vi "氨氮通讯.vi"() -> ()   [LabVIEW 2016, in "斯坦道氨氮.lvlib"]
uses:
  <vilib>/NI/Modbus Library/API/Wrapper/Create TCP Slave.vi
  <vilib>/Utility/config.llb/Write Key (String).vi
  <vilib>/Plasmionique/MB Master/MB_Master/MB_Master.lvclass
  <vilib>/NI/Modbus Library/API/slave/Modbus Slave.lvclass
  <vilib>/Utility/config.llb/NI_LVConfig.lvlib
  <vilib>/Plasmionique/MB Master/MB Master.lvlib
  <vilib>/NI/Modbus Library/API/Wrapper/API Main.lvlib
panel:
  out "测量数据区":T1 {"单位" items=["ug/L", "mg/L", "ppm", "mg/m3", "cm", "ppb", "ug/m3", "%", "nmol/mol", "umol/mol", "MPN/L", "MPN/100ml", "ng/m3", "NTU", "无量纲", "ms/cm", "us/cm", "℃", "mV", "万个/L"]}
  out "状态告警区":u16[](array[numeric])
  out "测量数据区":u16[](array[numeric])
  out "序列号":string
  out "状态告警区":T2 {"告警代码" items=["无告警", "缺试剂告警", "缺水样告警", "缺蒸馏水告警", "缺标液告警", "仪表漏液告警", "标定异常告警", "超量程告警", "加热异常", "低试剂预警", "超上限告警", "超下限告警", "仪表内部其他异常", "滴定异常告警", "电极异常告警", "量程切换告警", "参数设置告警", "PH电极电位异常", "电导率电极异常", "浊度光度异常", "溶解氧电极异常", "溶解氧光强异常", "温度异常告警", "PH异常告警", "溶解氧异常告警", "电导率异常告警", "浊度异常告警", "叶绿素异常告警", "藻密度异常告警", "蓝绿藻异常告警", "ORP异常告警", "氨氮异常告警", "清洁刷异常告警", "SD卡异常告警", "蓝牙异常告警", "Wifi异常告警", "流程异常告警"]; "故障代码" items=["无故障", "电机故障", "温度故障", "通讯故障", "滴定故障"]}
  out "status":bool
  out "关键参数区":T3
  in  "读关键参数区":bool
  in  "读状态告警区":bool
  in  "读测量数据区":bool
  in  "站号":u16(ring) items=["总磷"=1, "氨氮"=3]
  in  "停止":bool
  in  "启动":bool
  in  "控制命令":u16(ring) items=["启动测量"=1, "标样核查"=2, "零点核查"=3, "跨度核查"=4, "空白测试"=5, "平行样测试"=6, "加标回收"=7, "空白校准"=8, "标样校准"=9, "初始化（清洗）"=10, "停止测试"=11, "仪器重启"=12, "校时"=13, "模式设置"=14, "测量间隔设置"=15]
  in  "控制命令参数":u16[](array[numeric]) format="%04xH"
  in  "VISA Resource":refnum<visa-resource-name>
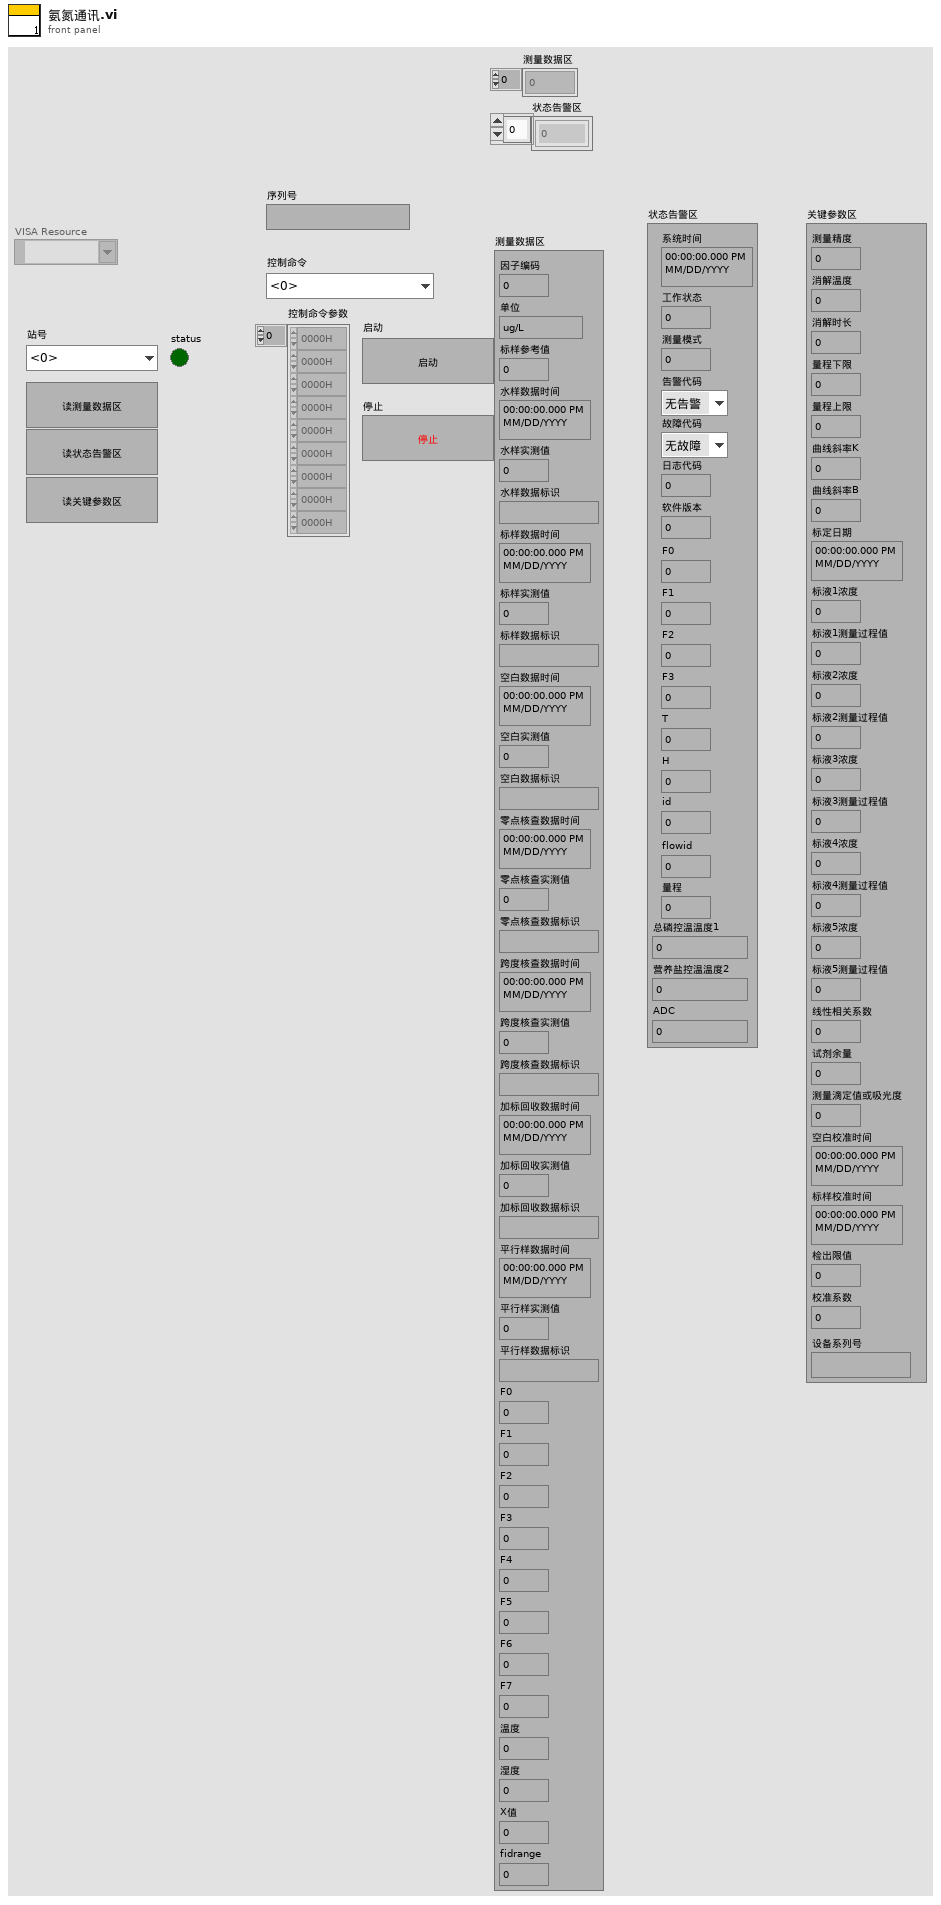
[diagram p1: front panel]
types:
  T1 = cluster{"因子编码":u32, "单位":u16, "标样参考值":sgl, "水样数据时间":timestamp, "水样实测值":sgl, "水样数据标识":string, "标样数据时间":timestamp, "标样实测值":sgl, "标样数据标识":string, "空白数据时间":timestamp, "空白实测值":sgl, "空白数据标识":string, "零点核查数据时间":timestamp, "零点核查实测值":sgl, "零点核查数据标识":string, "跨度核查数据时间":timestamp, "跨度核查实测值":sgl, "跨度核查数据标识":string, "加标回收数据时间":timestamp, "加标回收实测值":sgl, "加标回收数据标识":string, "平行样数据时间":timestamp, "平行样实测值":sgl, "平行样数据标识":string, "F0":sgl, "F1":sgl, "F2":sgl, "F3":sgl, "F4":sgl, "F5":sgl, "F6":sgl, "F7":sgl, "温度":sgl, "湿度":sgl, "X值":sgl, "fidrange":sgl}
  T2 = cluster{"系统时间":timestamp, "工作状态":u16, "测量模式":u16, "告警代码":u16, "故障代码":u16, "日志代码":u16, "软件版本":u16, "F0":sgl, "F1":sgl, "F2":sgl, "F3":sgl, "T":sgl, "H":sgl, "id":u16, "flowid":u16, "量程":u16, "ADC":sgl, "营养盐控温温度2":sgl, "总磷控温温度1":sgl}
  T3 = cluster{"测量精度":u16, "消解温度":u16, "消解时长":u16, "量程下限":sgl, "量程上限":sgl, "曲线斜率K":sgl, "曲线斜率B":sgl, "标定日期":timestamp, "标液1浓度":sgl, "标液1测量过程值":sgl, "标液2浓度":sgl, "标液2测量过程值":sgl, "标液3浓度":sgl, "标液3测量过程值":sgl, "标液4浓度":sgl, "标液4测量过程值":sgl, "标液5浓度":sgl, "标液5测量过程值":sgl, "线性相关系数":sgl, "试剂余量":u32, "测量滴定值或吸光度":sgl, "空白校准时间":timestamp, "标样校准时间":timestamp, "检出限值":sgl, "校准系数":sgl, "设备系列号":string}
  T4 = typedef "NI_LVConfig.lvlib/Config Data RefNum.ctl" = refnum<k1>
  T5 = enum8{"Enabled", "Disabled", "Disabled and Grayed Out"}
  T6 = cluster{"系统时间":timestamp, "工作状态":enum16{"空闲", "水样测试", "标样核查", "零点核查", "跨度核查", "空白测试", "平行样测试", "加标回收", "空白校准", "标样校准", "初始化（清洗）"}, "测量模式":enum16{"待机", "连续模式", "周期模式", "定点模式", "受控模式", "手动模式"}, "告警代码":u16, "故障代码":u16, "日志代码":u16, "软件版本":u16, "F0":sgl, "F1":sgl, "F2":sgl, "F3":sgl, "T":sgl, "H":sgl, "id":u16, "flowid":u16, "量程":u16, "总磷控温温度1":sgl, "营养盐控温温度2":sgl, "ADC":sgl}
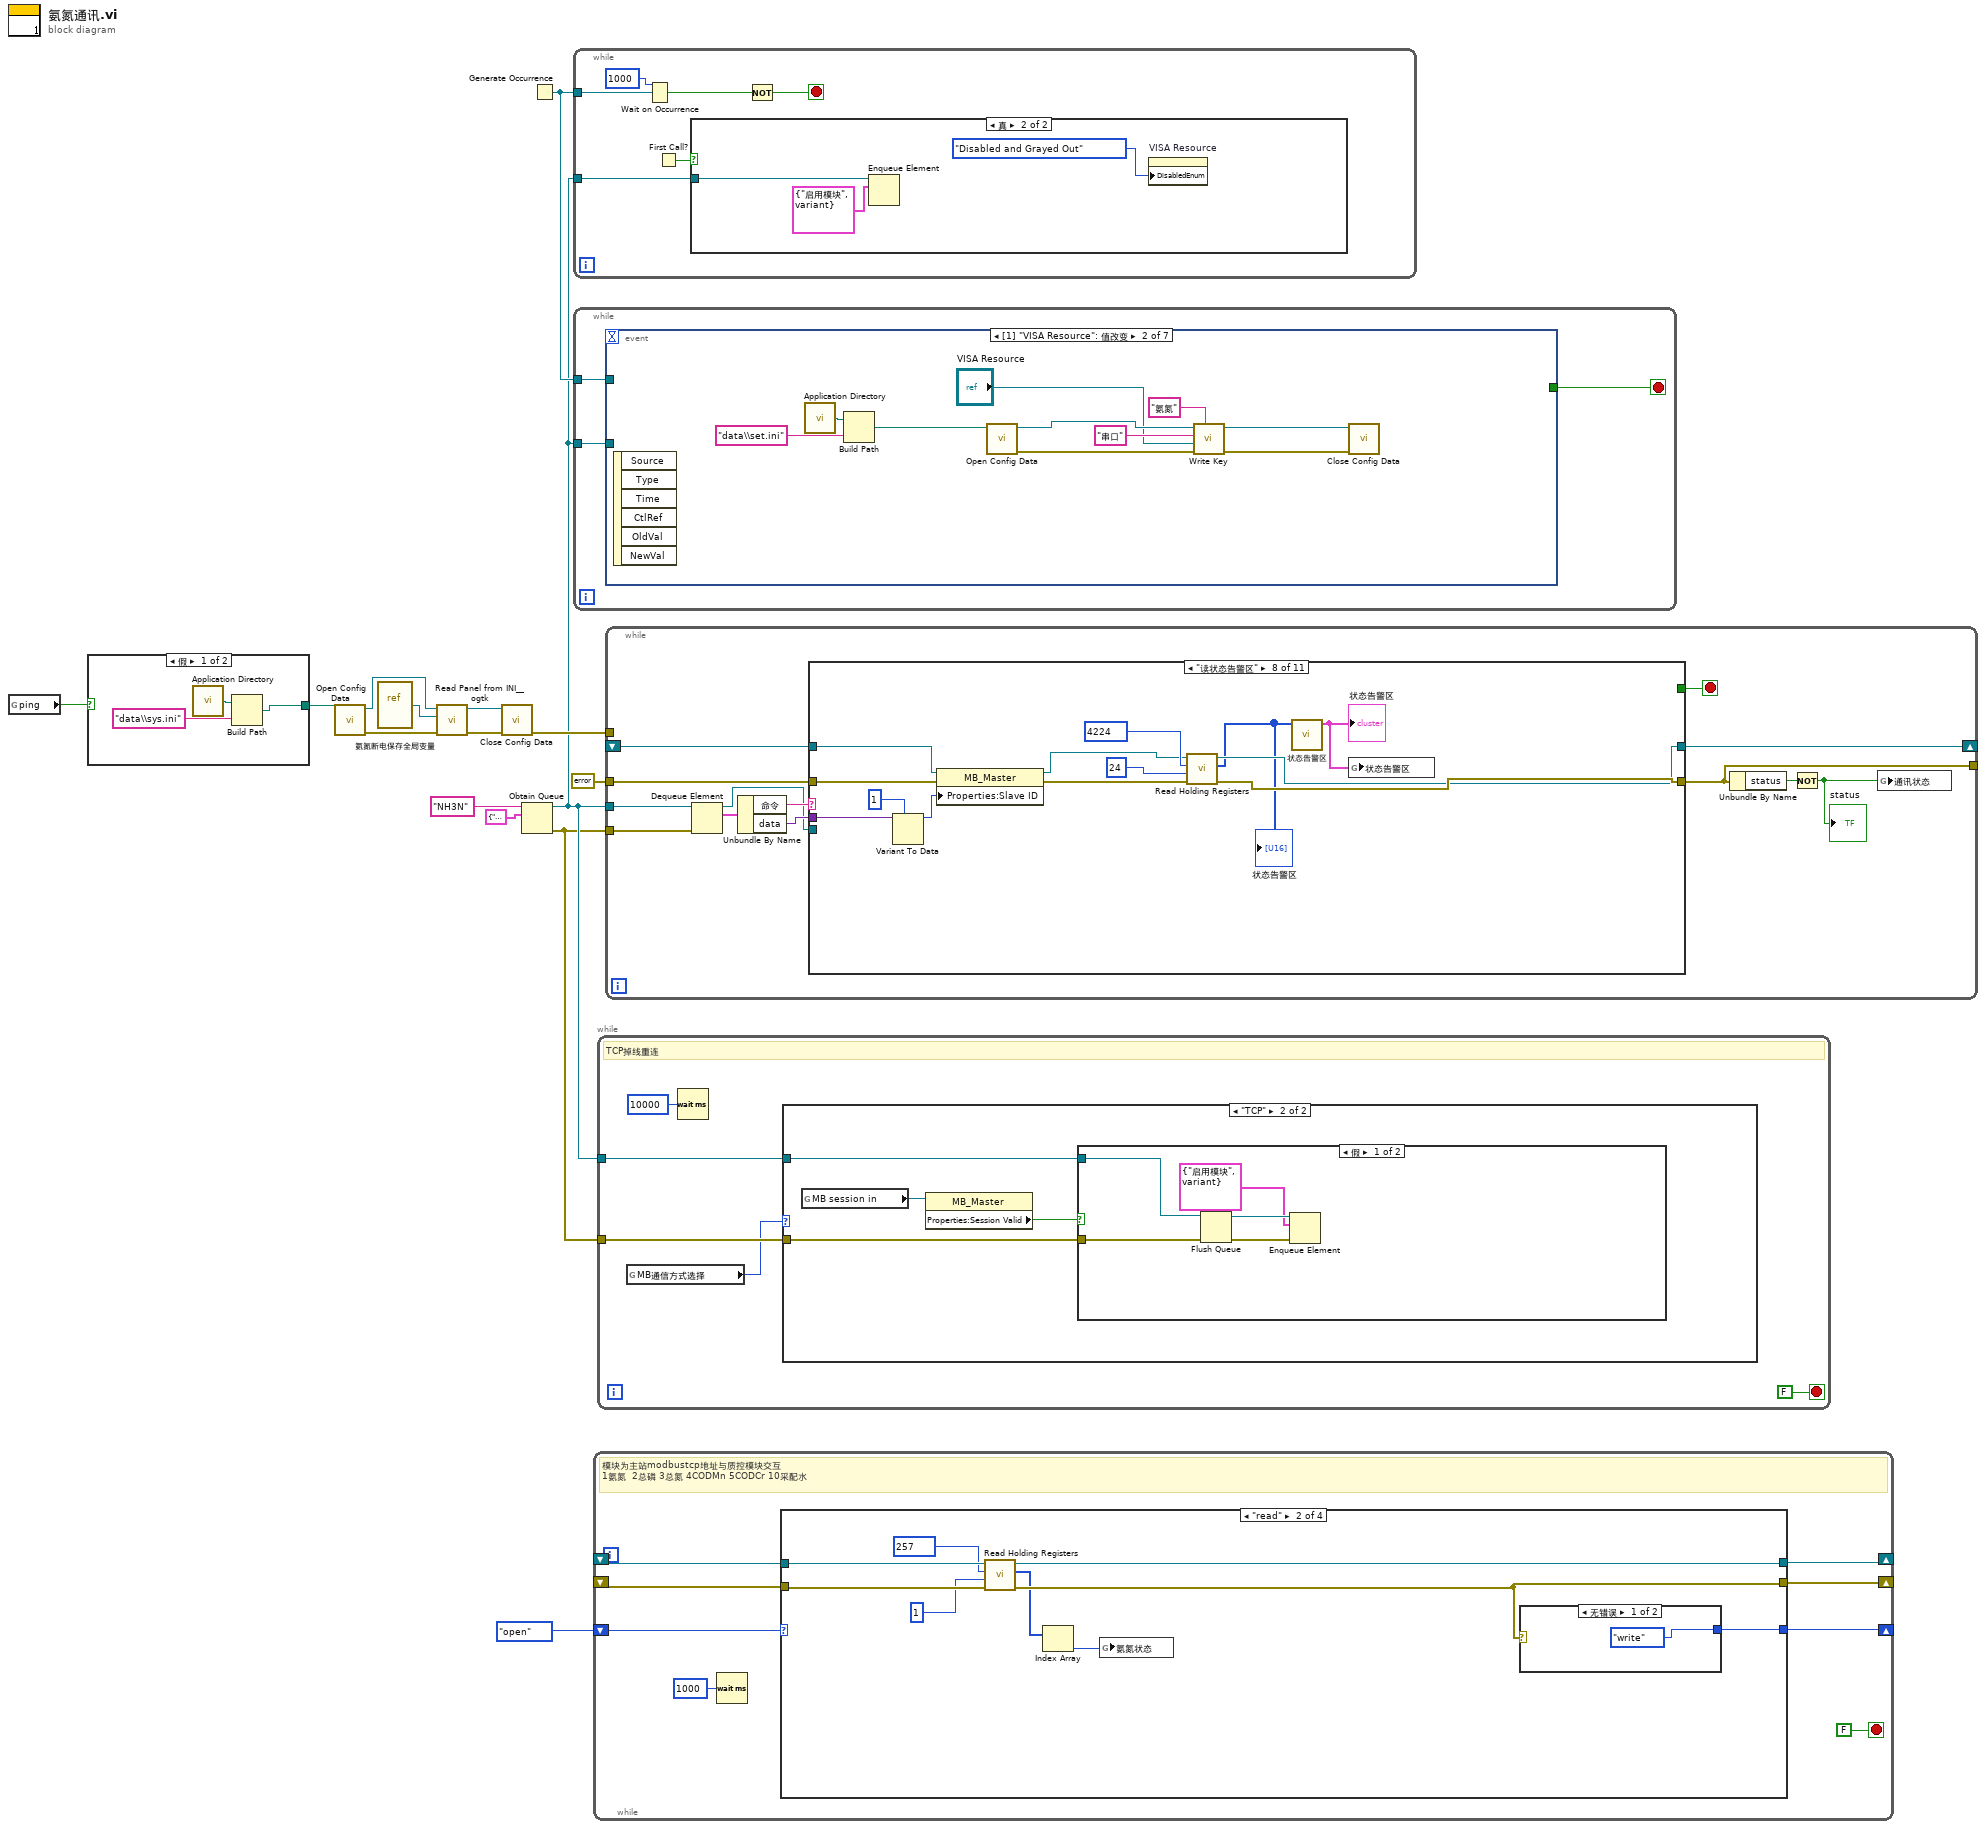
[diagram p0: block diagram]
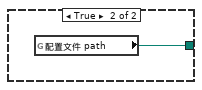
[diagram p2: hidden frame]
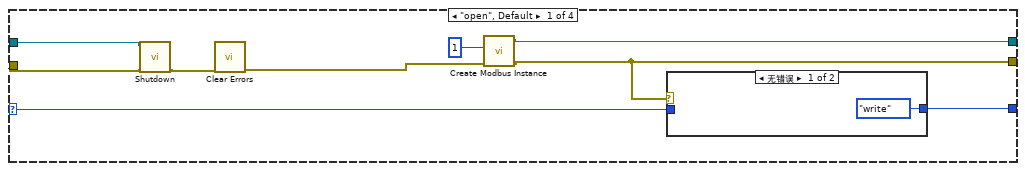
[diagram p5: hidden frame]
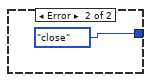
[diagram p7: hidden frame]
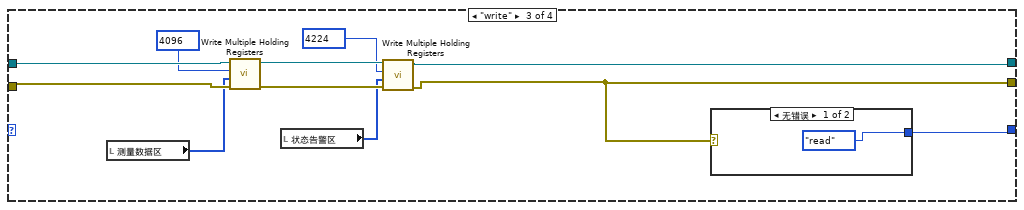
[diagram p8: hidden frame]
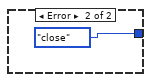
[diagram p9: hidden frame]
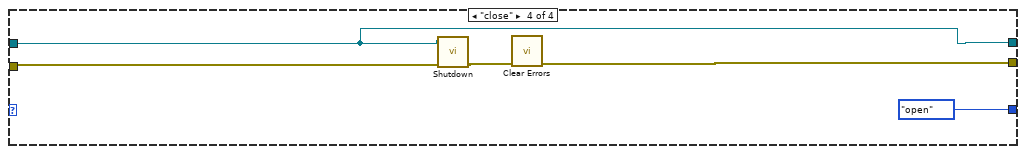
[diagram p10: hidden frame]
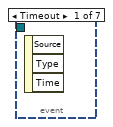
[diagram p12: hidden frame]
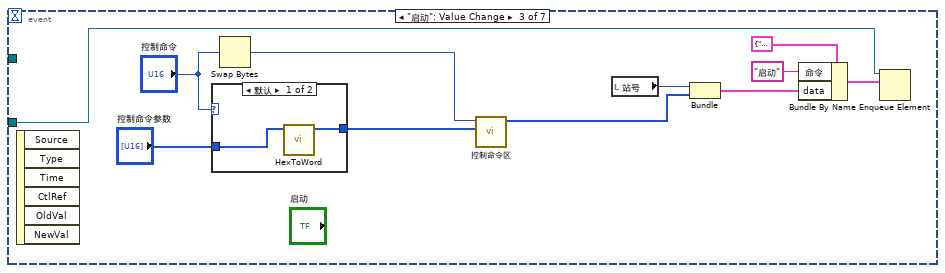
[diagram p13: hidden frame]
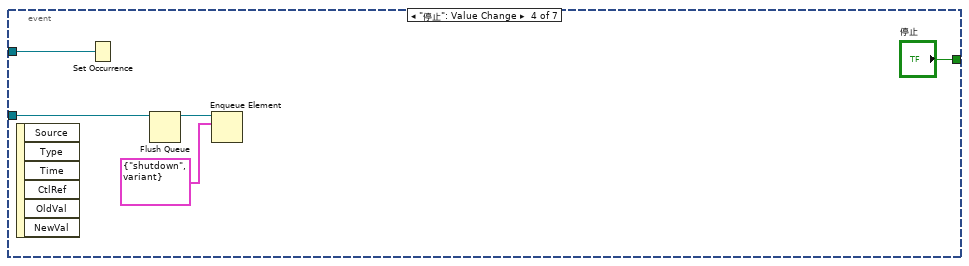
[diagram p15: hidden frame]
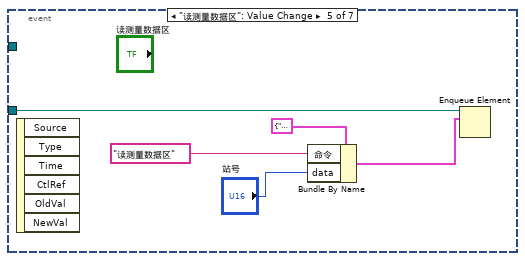
[diagram p16: hidden frame]
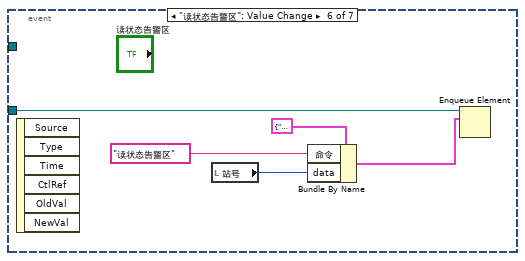
[diagram p17: hidden frame]
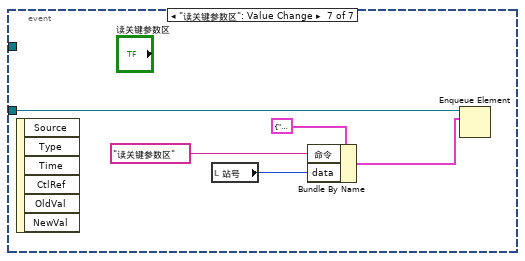
[diagram p18: hidden frame]
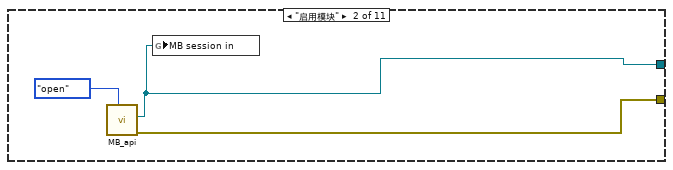
[diagram p20: hidden frame]
diagram:
  n1 = global read "VAR氨氮全局变量.vi" "ping"() -> (w2:bool)
  n2 = case shown="假" w2 {
    tunnel: [w16 w19] -> w1
    frame False {
      n3 = call <vilib>:"Application Directory.vi"() -> ("Application Directory"=w18:path)
      n4 = Build Path(base path=w18, name or relative path="data\\sys.ini" ("名称或相对路径")) -> (appended path=w16:path)
    }
    frame True {
      n5 = global read "VAR氨氮全局变量.vi" "配置文件 path"() -> (w19:path)
    }
  }
  n6 = call <vilib>:"Open Config Data.vi"("configuration file path"=w1) -> ("error out"=w10:errorcluster, "refnum"=w7:T4)  [unwired: 8 in, 1 out]
  n7 = vi-ref "氨氮断电保存全局变量.vi"() -> (w8:refnum<vi>)
  n8 = call <userlib>:"Read Panel from INI__ogtk.vi"("error in (no error)"=w10, "VI ref"=w8, "refnum"=w7) -> ("error out"=w11:errorcluster, "refnum out"=w9:T4)  [unwired: 7 in]
  n9 = call <vilib>:"Close Config Data.vi"("error in (no error)"=w11, "refnum"=w9) -> ("error out"=w6:errorcluster)  [unwired: 8 in, 1 out]
  n10 = Obtain Queue(name (unnamed)="NH3N" ("名称（未命名）"), element data type=cluster{"命令":string, "data":variant} {"命令"="", "data"=variant}) -> (queue out=w4:refnum<queue>, error out=w3:errorcluster)  [unwired: 3 in, 1 out]
  n11 = Generate Occurrence() -> (w12:refnum<k4>)
  n12 = while {
    tunnel: w12 -> [w25]
    tunnel: w4 -> [w21]
    stop <- w22 stop-if-true
    n13 = Wait on Occurrence(2:w25, 3:1000 ("毫秒超时(-1)")) -> (0:w23:bool)  [unwired: 1 in]
    n14 = First Call?() -> (First Call?: T/F=w20:bool)
    n15 = case shown="真" w20 {
      tunnel: w21 -> [_ w27]
      frame False {
      }
      frame True {
        n16 = Enqueue Element(queue=w27, element=cluster{"命令":string, "data":variant} {"命令"="启用模块", "data"=variant} ("元素")) -> ()  [unwired: 2 in, 3 out]
        n17 = property on="VISA Resource" class="VISAName"("DisabledEnum"=T5."Disabled and Grayed Out" ("禁用")) -> ()  [unwired: 2 in, 2 out]
      }
    }
    n18 = Not(x=w23) -> (.not. x?=w22:bool)
  }
  n19 = while {
    tunnel: w4 -> [w31]
    tunnel: w12 -> [w29]
    stop <- w30 stop-if-true
    n20 = event shown="[1] \"VISA Resource\": 值改变" {
      selector: _ -> [_ _ _ _ _ _ _]
      dyn-events: _ -> [_ _ _ _ _ _ _]
      timeout: _ -> [_ _ _ _ _ _ _]
      tunnel: w31 -> [_ _ w52 w59 w65 w70 w75]
      tunnel: [_ _ _ "停止" _ _ _] -> w30
      tunnel: w29 -> [_ _ _ w56 _ _ _]
      event Timeout {
        n21 = event-data() -> ()  [unwired: 1 in, 3 out]
      }
      event "VISA Resource": Value Change {
        n22 = event-data() -> ()  [unwired: 1 in, 6 out]
        n23 = call <vilib>:"Application Directory.vi"() -> ("Application Directory"=w34:path)
        n24 = Build Path(base path=w34, name or relative path="data\\set.ini" ("名称或相对路径")) -> (appended path=w35:path)
        n25 = call <vilib>:"Open Config Data.vi"("configuration file path"=w35) -> ("error out"=w41:errorcluster, "refnum"=w40:T4)  [unwired: 8 in, 1 out]
        n26 = call-poly <vilib>:"Write Key.vi"("section"="氨氮", "error in (no error)"=w41, "value"="VISA Resource", "key"="串口", "refnum"=w40) -> ("error out"=w37:errorcluster, "refnum out"=w33:T4)  [unwired: 4 in, 1 out]
        n27 = call <vilib>:"Close Config Data.vi"("error in (no error)"=w37, "refnum"=w33) -> ()  [unwired: 8 in, 2 out]
      }
      event "启动": Value Change {
        n28 = event-data() -> ()  [unwired: 1 in, 6 out]
        n29 = case shown="默认" "控制命令" {
          tunnel: "控制命令参数" -> [w54 w55]
          tunnel: [w53 w55] -> w42
          frame Default {
            n30 = call "HexToWord.vi"("数组"=w54) -> ("WORD"=w53:u16[])  [unwired: 10 in]
          }
          frame 13 {
          }
        }
        n31 = Swap Bytes(anything="控制命令") -> (byte swapped=w45:u16)
        n32 = call "控制命令区.vi"("控制命令参数"=w42, "控制命令"=w45) -> ("控制命令"=w48:u16[])  [unwired: 9 in]
        n33 = local read "站号"() -> (w47:u16)
        n34 = Bundle("站号"=w47, "控制命令"=w48) -> (w46:cluster{"站号":u16, "控制命令":u16[]})  [unwired: 1 in]
        n35 = Bundle By Name(cluster=cluster{"命令":string, "data":variant} {"命令"="", "data"=variant} ("元素"), "命令"="启动", "data"=w46) -> (w50:cluster{"命令":string, "data":variant})
        n36 = Enqueue Element(queue=w52, element=w50) -> ()  [unwired: 2 in, 3 out]
      }
      event "停止": Value Change {
        n37 = event-data() -> ()  [unwired: 1 in, 6 out]
        n38 = Set Occurrence(w56) -> ()
        n39 = Flush Queue(queue=w59) -> (queue out=w58:refnum<queue>)  [unwired: 1 in, 2 out]
        n40 = Enqueue Element(queue=w58, element=cluster{"命令":string, "data":variant} {"命令"="shutdown", "data"=variant} ("元素")) -> ()  [unwired: 2 in, 3 out]
      }
      event "读测量数据区": Value Change {
        n41 = event-data() -> ()  [unwired: 1 in, 6 out]
        n42 = Bundle By Name(cluster=cluster{"命令":string, "data":variant} {"命令"="", "data"=variant} ("元素"), "命令"="读测量数据区", "data"="站号") -> (w63:cluster{"命令":string, "data":variant})
        n43 = Enqueue Element(queue=w65, element=w63) -> ()  [unwired: 2 in, 3 out]
      }
      event "读状态告警区": Value Change {
        n44 = event-data() -> ()  [unwired: 1 in, 6 out]
        n45 = local read "站号"() -> (w66:u16)
        n46 = Bundle By Name(cluster=cluster{"命令":string, "data":variant} {"命令"="", "data"=variant} ("元素"), "命令"="读状态告警区", "data"=w66) -> (w68:cluster{"命令":string, "data":variant})
        n47 = Enqueue Element(queue=w70, element=w68) -> ()  [unwired: 2 in, 3 out]
      }
      event "读关键参数区": Value Change {
        n48 = event-data() -> ()  [unwired: 1 in, 6 out]
        n49 = local read "站号"() -> (w71:u16)
        n50 = Bundle By Name(cluster=cluster{"命令":string, "data":variant} {"命令"="", "data"=variant} ("元素"), "命令"="读关键参数区", "data"=w71) -> (w73:cluster{"命令":string, "data":variant})
        n51 = Enqueue Element(queue=w75, element=w73) -> ()  [unwired: 2 in, 3 out]
      }
    }
  }
  n52 = while {
    shift-right: [w81] -> _
    shift-left: _ -> [w83]
    shift-right: [w80] -> _
    shift-left: _ -> [w82]
    shift-right: [w77] -> _
    shift-left: enum16{"open", "read", "write", "close"}."open" -> [w78]
    stop <- FALSE stop-if-true
    # "模块为主站modbustcp地址与质控模块交互\n1氨氮  2总磷 3总氮 4CODMn 5CODCr 10采配水"
    n53 = Wait (ms)(milliseconds to wait=u32 1000 ("等待时间（毫秒）")) -> ()  [unwired: 1 out]
    n54 = case shown="\"read\"" w78 {
      selector: w78 -> [w92 _ _ _]
      tunnel: w83 -> [w86 w102 w115 w121]
      tunnel: w82 -> [w85 w100 w114 w120]
      tunnel: [w89 w101 w110 w121] -> w81
      tunnel: [w88 w99 w109 w123] -> w80
      tunnel: [w91 w103 w116 enum16{"open", "read", "write", "close"}."open"] -> w77
      frame "open", Default {
        n55 = call-dynamic "Shutdown.vi"("error in"=w85, "Modbus slave in"=w86) -> ("error out"=w84:errorcluster)  [unwired: 9 in]
        n56 = call <vilib>:"Clear Errors.vi"("error in (no error)"=w84) -> ("error out"=w87:errorcluster)  [unwired: 5 in, 1 out]
        n57 = call-poly <vilib>:"Create Modbus Instance.vi"("error in"=w87, "port (502)"=u16 1) -> ("error out"=w88:errorcluster, "TCP slave instance"=w89:refnum<class "Modbus Slave.lvclass">)  [unwired: 8 in]
        n58 = case shown="无错误" w88 {
          tunnel: w92 -> [_ w94]
          tunnel: [enum16{"open", "read", "write", "close"}."write" w94] -> w91
          frame No Error {
          }
          frame Error {
          }
        }
      }
      frame "read" {
        n59 = call-dynamic <vilib>:"Read Holding Registers.vi"("error in"=w100, "number of inputs"=u16 1, "starting address"=u16 257, "Modbus slave in"=w102) -> ("error out"=w99:errorcluster, "register values"=w96:u16[], "Modbus slave out"=w101:refnum<class "Modbus Slave.lvclass">)  [unwired: 5 in]
        n60 = Index Array(array=w96) -> (element=w95:u16)  [unwired: 1 in]
        n61 = global write "VAR氨氮全局变量.vi" "氨氮状态"(w95) -> ()
        n62 = case shown="无错误" w99 {
          tunnel: [enum16{"open", "read", "write", "close"}."write" enum16{"open", "read", "write", "close"}."close"] -> w103
          frame No Error {
          }
          frame Error {
          }
        }
      }
      frame "write" {
        n63 = local read "测量数据区"() -> (w108:u16[])
        n64 = call-dynamic "Write Multiple Holding Registers.vi"("error in"=w114, "registers to write"=w108, "starting address"=u16 4096, "Modbus slave in"=w115) -> ("error out"=w111:errorcluster, "Modbus slave out"=w112:refnum<class "Modbus Slave.lvclass">)  [unwired: 6 in]
        n65 = local read "状态告警区"() -> (w106:u16[])
        n66 = call-dynamic "Write Multiple Holding Registers.vi"("error in"=w111, "registers to write"=w106, "starting address"=u16 4224, "Modbus slave in"=w112) -> ("error out"=w109:errorcluster, "Modbus slave out"=w110:refnum<class "Modbus Slave.lvclass">)  [unwired: 6 in]
        n67 = case shown="无错误" w109 {
          tunnel: [enum16{"open", "read", "write", "close"}."read" enum16{"open", "read", "write", "close"}."close"] -> w116
          frame No Error {
          }
          frame Error {
          }
        }
      }
      frame "close" {
        n68 = call-dynamic "Shutdown.vi"("error in"=w120, "Modbus slave in"=w121) -> ("error out"=w119:errorcluster)  [unwired: 9 in]
        n69 = call <vilib>:"Clear Errors.vi"("error in (no error)"=w119) -> ("error out"=w123:errorcluster)  [unwired: 5 in, 1 out]
      }
    }
  }
  n70 = while "While循环" {
    tunnel: w4 -> [w126]
    tunnel: w3 -> [w125]
    stop <- FALSE stop-if-true
    # "TCP掉线重连"
    n71 = global read "氨氮断电保存全局变量.vi" "MB通信方式选择"() -> (w124:enum16{"串口", "TCP"})
    n72 = Wait (ms)(milliseconds to wait=u32 10000 ("等待时间（毫秒）")) -> ()  [unwired: 1 out]
    n73 = case shown="\"TCP\"" w124 {
      tunnel: w126 -> [_ w131]
      tunnel: w125 -> [_ w130]
      frame "串口", Default {
      }
      frame "TCP" {
        n74 = global read "VAR氨氮全局变量.vi" "MB session in"() -> (w129:refnum<class "MB_Master.lvclass">)
        n75 = property class="MB_Master"(reference=w129) -> ("Properties:Session Valid"=w132:bool)  [unwired: 1 in, 2 out]
        n76 = case shown="假" w132 {
          tunnel: w131 -> [w135 _]
          tunnel: w130 -> [w134 _]
          frame False {
            n77 = Flush Queue(queue=w135, error in (no error)=w134) -> (queue out=w137:refnum<queue>, error out=w136:errorcluster)  [unwired: 1 out]
            n78 = Enqueue Element(queue=w137, element=cluster{"命令":string, "data":variant} {"命令"="启用模块", "data"=variant} ("元素"), error in (no error)=w136) -> ()  [unwired: 1 in, 3 out]
          }
          frame True {
          }
        }
      }
    }
  }
  n79 = while {
    tunnel: w4 -> [w150]
    tunnel: w3 -> [w149]
    shift-right: [w147] -> _
    shift-left: _ -> [w146]
    tunnel: errorcluster {"status"=FALSE, "code"=0, "source"=""} ("error out") -> [w145]
    tunnel: [w140] -> _
    tunnel: w6 -> [_]
    stop <- w148 stop-if-true
    n80 = Dequeue Element(queue=w150, error in (no error)=w149) -> (queue out=w141:refnum<queue>, element=w143:cluster{"命令":string, "data":variant})  [unwired: 1 in, 2 out]
    n81 = Unbundle By Name(w143) -> ("命令"=w144:string, "data"=w142:variant)
    n82 = case shown="\"读状态告警区\"" w144 {
      tunnel: w142 -> [_ _ _ w169 w180 w197 w206 w216 w231 w245 _]
      tunnel: w141 -> [_ _ _ _ _ _ _ _ _ _ w258]
      tunnel: [_ _ _ _ _ _ _ _ _ _ TRUE] -> w148
      tunnel: [w151 w154 w156 w172 w183 w199 w211 w225 w238 w252 w254] -> w147
      tunnel: [w152 w153 w157 w171 w182 w198 w200 w226 w239 w253 w255] -> w140
      tunnel: w146 -> [w151 _ w156 w168 w179 w196 w205 w219 w234 w248 w254]
      tunnel: w145 -> [w152 _ w159 w165 w176 w193 w203 w220 w235 w249 w256]
      frame Default {
      }
      frame "启用模块" {
        n83 = call "MB_api.vi"("STEP"=enum16{"open", "read", "write", "close"}."open") -> ("error out"=w153:errorcluster, "MB session out"=w154:refnum<class "MB_Master.lvclass">)  [unwired: 8 in, 1 out]
        n84 = global write "VAR氨氮全局变量.vi" "MB session in"(w154) -> ()
      }
      frame "停用模块" {
        n85 = call-dynamic "Close Session.vi"("error in (no error)"=w159, "MB session in"=w156) -> ("error out"=w158:errorcluster)  [unwired: 9 in]
        n86 = call <vilib>:"Clear Errors.vi"("error in (no error)"=w158) -> ("error out"=w157:errorcluster)  [unwired: 5 in, 1 out]
      }
      frame "启动" {
        n87 = Variant To Data(type=cluster{"站号":u16, "控制命令":u16[]} {"站号"=0, "控制命令"=[]} ("输出簇"), Variant=w169) -> (data=w163:cluster{"站号":u16, "控制命令":u16[]})  [unwired: 1 in, 1 out]
        n88 = Unbundle By Name(w163) -> ("站号"=w162:u16, "控制命令"=w160:u16[])
        n89 = property class="MB_Master"(reference=w168, error in=w165, "Properties:Slave ID"=w162) -> (reference out=w167:refnum<class "MB_Master.lvclass">, error out=w166:errorcluster)
        n90 = Index Array(array=w160) -> (element=w161:u16)  [unwired: 1 in]
        n91 = global write "VAR氨氮全局变量.vi" "控制命令"(w161) -> ()
        n92 = call <vilib>:"Write Multiple Registers.vi"("error in (no error)"=w166, "values"=w160, "starting address"=u16 4608, "MB session in"=w167) -> ("error out"=w171:errorcluster, "MB session out"=w172:refnum<class "MB_Master.lvclass">)  [unwired: 6 in]
      }
      frame "盲样测试" {
        n93 = Variant To Data(type=0, Variant=w180) -> (data=w173:i32)  [unwired: 1 in, 1 out]
        n94 = property class="MB_Master"(reference=w179, error in=w176, "Properties:Slave ID"=w173) -> (reference out=w178:refnum<class "MB_Master.lvclass">, error out=w177:errorcluster)
        n95 = case shown="默认" w173 {
          tunnel: [u16[] [] ("values") u16[] [33539, 0] ("values") u16[] [23555, 0] ("values")] -> w175
          frame Default {
          }
          frame 1 {
            # "总磷盲样测试命令"
          }
          frame 3 {
            # "氨氮盲样测试"
          }
        }
        n96 = call <vilib>:"Write Multiple Registers.vi"("error in (no error)"=w177, "values"=w175, "starting address"=u16 24592, "MB session in"=w178) -> ("error out"=w182:errorcluster, "MB session out"=w183:refnum<class "MB_Master.lvclass">)  [unwired: 6 in]
      }
      frame "debug" {
        n97 = Variant To Data(type=cluster{"站号":u16, "控制命令":u16[]} {"站号"=0, "控制命令"=[]} ("输出簇"), Variant=w197) -> (data=w191:cluster{"站号":u16, "控制命令":u16[]})  [unwired: 1 in, 1 out]
        n98 = Unbundle By Name(w191) -> ("站号"=w190:u16, "控制命令"=w188:u16[])
        n99 = property class="MB_Master"(reference=w196, error in=w193, "Properties:Slave ID"=w190) -> (reference out=w195:refnum<class "MB_Master.lvclass">, error out=w194:errorcluster)
        n100 = Index Array(array=w188) -> (element=w189:u16)  [unwired: 1 in]
        n101 = global write "VAR氨氮全局变量.vi" "控制命令"(w189) -> ()
        n102 = call <vilib>:"Write Multiple Registers.vi"("error in (no error)"=w194, "values"=w188, "starting address"=u16 24594, "MB session in"=w195) -> ("error out"=w198:errorcluster, "MB session out"=w199:refnum<class "MB_Master.lvclass">)  [unwired: 6 in]
      }
      frame "读测量数据区" {
        n103 = Variant To Data(type=u8 1 ("Slave ID"), Variant=w206) -> (data=w207:u8)  [unwired: 1 in, 1 out]
        n104 = property class="MB_Master"(reference=w205, error in=w203, "Properties:Slave ID"=w207) -> (reference out=w204:refnum<class "MB_Master.lvclass">, error out=w202:errorcluster)
        n105 = call <vilib>:"Read Holding Registers.vi"("error in (no error)"=w202, "quantity"=u16 105, "starting address"=u16 4096, "MB session in"=w204) -> ("error out"=w200:errorcluster, "Registers"=w201:u16[], "MB session out"=w211:refnum<class "MB_Master.lvclass">)  [unwired: 5 in]
        n106 = case shown="无错误" w200 {
          tunnel: w201 -> [w213 _]
          frame No Error {
            n107 = call "测量数据区.vi"("数组"=w213) -> ("测量数据区"=w212:T1)  [unwired: 10 in]
            "测量数据区" <- w212
            n108 = global write "VAR氨氮全局变量.vi" "测量数据区"(w212) -> ()
            "测量数据区" <- w213
          }
          frame Error {
          }
        }
      }
      frame "读状态告警区" {
        n109 = Variant To Data(type=u8 1 ("Slave ID"), Variant=w216) -> (data=w221:u8)  [unwired: 1 in, 1 out]
        n110 = property class="MB_Master"(reference=w219, error in=w220, "Properties:Slave ID"=w221) -> (reference out=w218:refnum<class "MB_Master.lvclass">, error out=w217:errorcluster)
        n111 = call <vilib>:"Read Holding Registers.vi"("error in (no error)"=w217, "quantity"=u16 24, "starting address"=u16 4224, "MB session in"=w218) -> ("error out"=w226:errorcluster, "Registers"=w215:u16[], "MB session out"=w225:refnum<class "MB_Master.lvclass">)  [unwired: 5 in]
        "状态告警区" <- w215
        n112 = call "状态告警区.vi"("数组"=w215) -> ("状态告警区"=w214:T6)  [unwired: 10 in]
        "状态告警区" <- w214
        n113 = global write "VAR氨氮全局变量.vi" "状态告警区"(w214) -> ()
      }
      frame "读关键参数区" {
        n114 = Variant To Data(type=u8 1 ("Slave ID"), Variant=w231) -> (data=w229:u8)  [unwired: 1 in, 1 out]
        n115 = property class="MB_Master"(reference=w234, error in=w235, "Properties:Slave ID"=w229) -> (reference out=w233:refnum<class "MB_Master.lvclass">, error out=w232:errorcluster)
        n116 = call <vilib>:"Read Holding Registers.vi"("error in (no error)"=w232, "quantity"=u16 19, "starting address"=u16 4256, "MB session in"=w233) -> ("error out"=w239:errorcluster, "Registers"=w228:u16[], "MB session out"=w238:refnum<class "MB_Master.lvclass">)  [unwired: 5 in]
        n117 = call "关键参数区.vi"("数组"=w228) -> ("关键参数区"=w227:T3)  [unwired: 10 in]
        "关键参数区" <- w227
        n118 = global write "VAR氨氮全局变量.vi" "关键参数区"(w227) -> ()
      }
      frame "读序列号" {
        n119 = Variant To Data(type=u8 1 ("Slave ID"), Variant=w245) -> (data=w243:u8)  [unwired: 1 in, 1 out]
        n120 = property class="MB_Master"(reference=w248, error in=w249, "Properties:Slave ID"=w243) -> (reference out=w247:refnum<class "MB_Master.lvclass">, error out=w246:errorcluster)
        n121 = call <vilib>:"Read Holding Registers.vi"("error in (no error)"=w246, "quantity"=u16 6, "starting address"=u16 4, "MB session in"=w247) -> ("error out"=w253:errorcluster, "Registers"=w242:u16[], "MB session out"=w252:refnum<class "MB_Master.lvclass">)  [unwired: 5 in]
        n122 = call "HexToString.vi"("数组"=w242) -> ("STRING"=w241:string[])  [unwired: 10 in]
        n123 = Index Array(array=w241) -> (element=w240:string)  [unwired: 1 in]
        "序列号" <- w240
        n124 = global write "VAR氨氮全局变量.vi" "序列号"(w240) -> ()
      }
      frame "shutdown" {
        n125 = call-dynamic "Close Session.vi"("error in (no error)"=w256, "MB session in"=w254) -> ("error out"=w255:errorcluster)  [unwired: 9 in]
        n126 = Flush Queue(queue=w258) -> (queue out=w257:refnum<queue>)  [unwired: 1 in, 2 out]
        n127 = Release Queue(queue=w257) -> ()  [unwired: 2 in, 3 out]
      }
    }
    n128 = Unbundle By Name(w140) -> ("status"=w139:bool)
    n129 = Not(x=w139) -> (.not. x?=w138:bool)
    "status" <- w138
    n130 = global write "VAR氨氮全局变量.vi" "通讯状态"(w138) -> ()
  }
